vi "HarvestPips.vi"(7 "BananaPeel in":refnum<class "BananaPeel.lvclass">, 11 "Pips":refnum<class "Pips.lvclass">) -> (0 "error out":errorcluster, 3 "Pips":refnum<class "Pips.lvclass">)   [LabVIEW 2021, in "Bananas.lvlib" / "BananaPeel.lvclass"]
uses:
  BananaPeel.lvclass
  Pips/Pips.lvclass
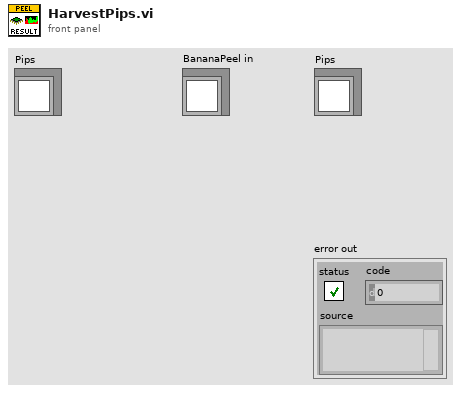
[diagram p1: front panel]
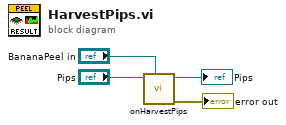
[diagram p0: block diagram]
diagram:
  n1 = call-dynamic "onHarvestPips.vi"("BananaPeel in"="BananaPeel in", "Pips"="Pips") -> ("error out"=→"error out":errorcluster, "Pips"=→"Pips":refnum<class "Pips.lvclass">)  [unwired: 8 in]
